vi "Keithley2612b_IV LOOP.vi"(3 "Error Query (False)":bool, 4 "Limit":dbl=1.0, 7 "Source Function (Current)":enum32{"Current", "Voltage"}(ring)=enum."Voltage", 8 "error in (no error)":errorcluster, 9 "Channel (Channel A)":T1, 10 "Node (0-64)":i8 min=0 max=64 step=1, 11 "VISA resource name":refnum<visa-resource-name>) -> (0 "error out":errorcluster)   [LabVIEW 2016]
doc: "This example shows how to configure the source and take a measurement."
uses:
  <instrlib>/Keithley 2600 Series/Public/Channel.ctl
  <vilib>/express/express shared/transition.llb/Dynamic To Waveform Array.vi
  <vilib>/express/express signal manip/GetorSetDDTAttributes/Set DDT Attributes/SetT0.vi
  <vilib>/express/express shared/transition.llb/Waveform Array To Dynamic.vi
  <vilib>/express/express signal manip/GetorSetDDTAttributes/Set DDT Attributes/Set DDT Properties.xnode
  <instrlib>/Keithley 2600 Series/Keithley 2600 Series.lvlib
panel:
  out "Current Number Past":dbl
  out "Voltage Output":string
  out "Current Output":string
  in  "Delay (s)":dbl
  in  "Step Size":dbl
  in  "End Voltage":dbl
  in  "Start Voltage":dbl
  # "(c) 2008 Keithley Instruments, Inc.  ALL RIGHTS RESERVED."
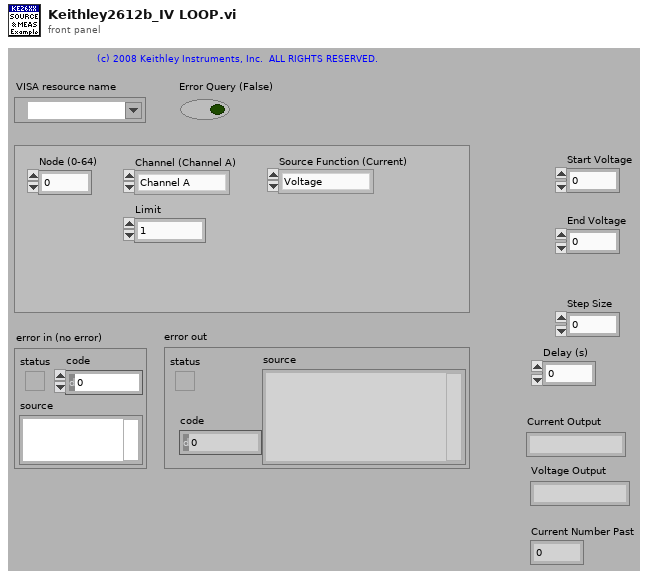
[diagram p1: front panel]
types:
  T1 = typedef "Keithley 2600 Series.lvlib/Channel.ctl" = enum32{"Channel A", "Channel B"}
  T2 = typedef "NI_Matrix.lvlib/RealMatrix.ctl" = dbl[][]
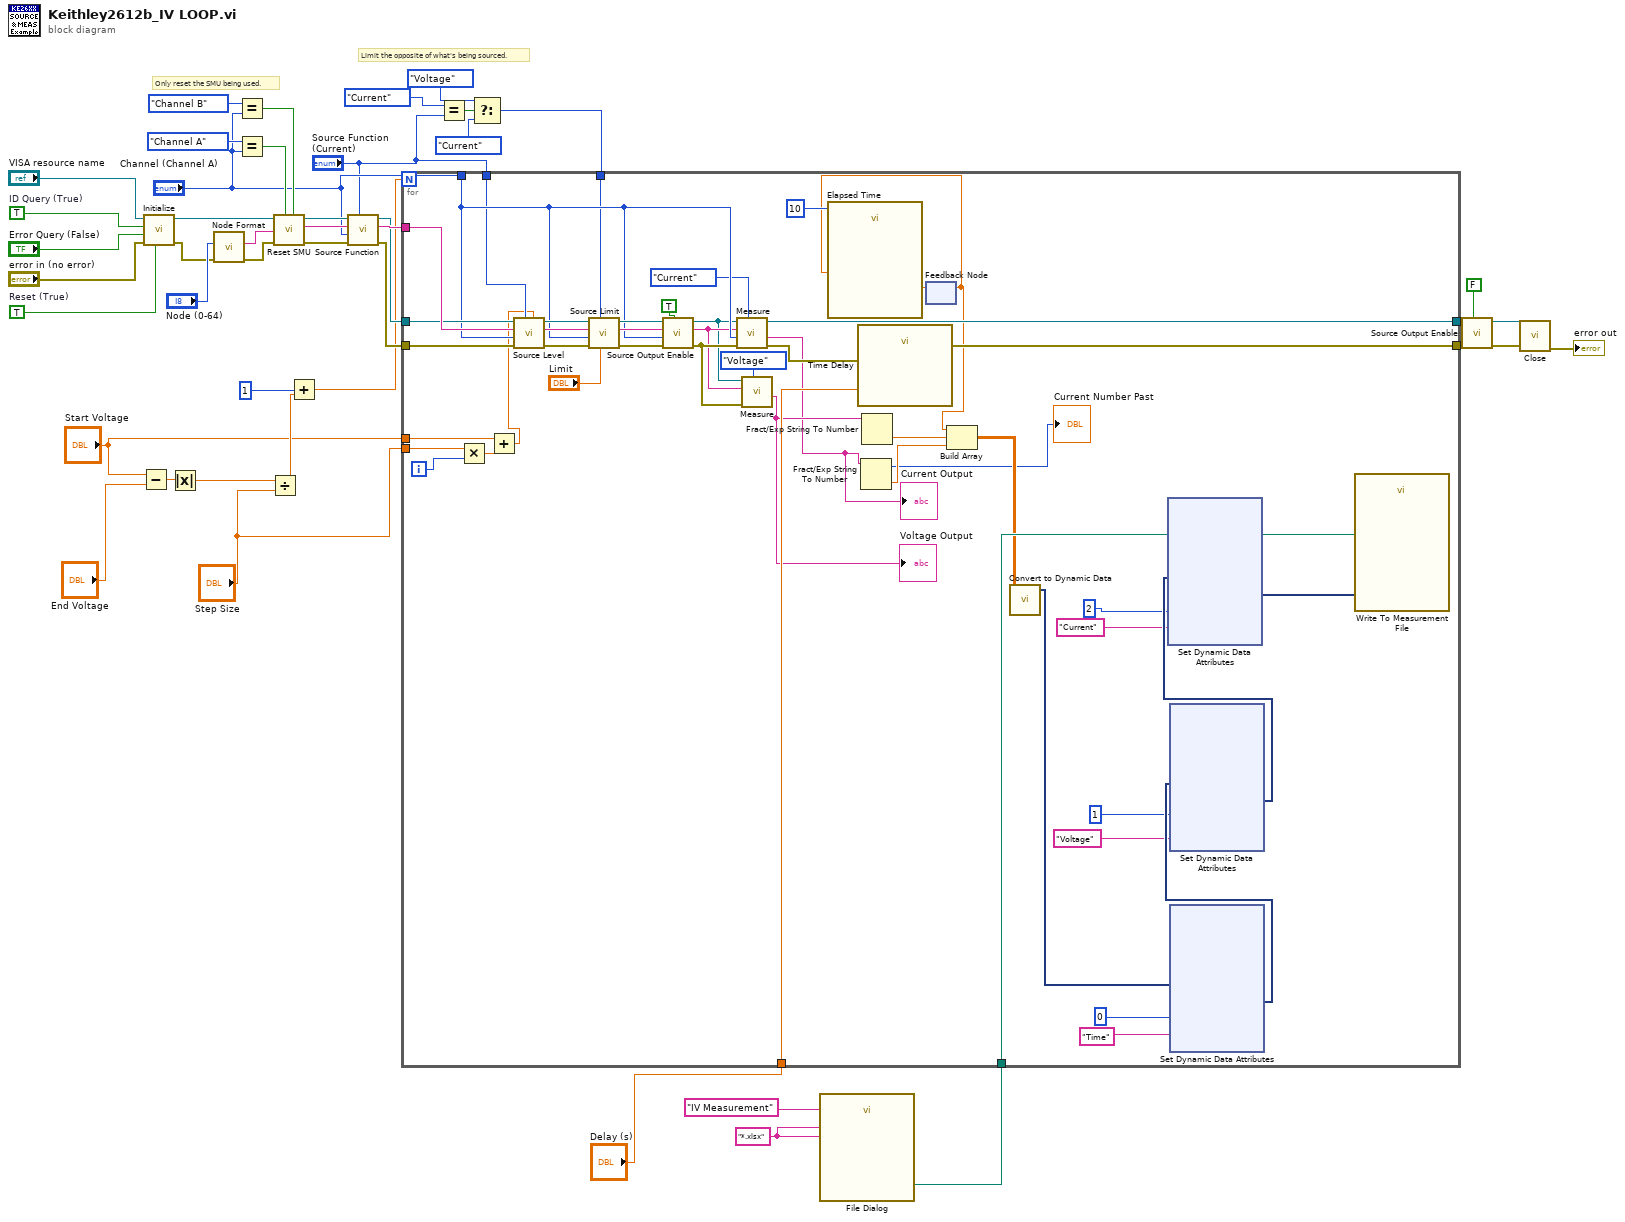
[diagram p0: block diagram]
diagram:
  w11 = "*.xlsx"
  w32 = TRUE  # Reset (True)
  w43 = TRUE  # ID Query (True)
  # "Limit the opposite of what's being sourced."
  # "Only reset the SMU being used."
  n1 = Subtract(x="Start Voltage", y="End Voltage") -> (x-y=w8:dbl)
  n2 = call <instrlib>:"Initialize.vi"("Reset (True)"=w32, "error in (no error)"="error in (no error)", "Error Query (False)"="Error Query (False)", "ID Query (True)"=w43, "VISA resource name"="VISA resource name") -> ("error out"=w1:errorcluster, "VISA resource name out"=w41:refnum<visa-resource-name>)  [unwired: 1 in, 4 out]
  n3 = Absolute Value(x=w8) -> (abs(x)=w7:dbl)
  n4 = call <instrlib>:"Node Format.vi"("error in"=w1, "Node (0-64)"="Node (0-64)") -> ("error out"=w28:errorcluster, "Formatted Node"=w29:string)  [unwired: 8 out]
  n5 = Equal?(x=enum32{"Channel A", "Channel B"}."Channel B", y="Channel (Channel A)") -> (x = y?=w37:bool)
  n6 = Equal?(x=enum32{"Channel A", "Channel B"}."Channel A", y="Channel (Channel A)") -> (x = y?=w38:bool)
  n7 = Divide(x=w7, y="Step Size") -> (x/y=w5:dbl)
  n8 = call <instrlib>:"Reset SMU.vi"("SMU B (No)"=w37, "SMU A (No)"=w38, "error in (no error)"=w28, "Node In"=w29, "VISA resource name"=w41) -> ("error out"=w36:errorcluster, "Node Out"=w34:string, "VISA resource name out"=w35:refnum<visa-resource-name>)  [unwired: 4 out]
  n9 = Add(x=1, y=w5) -> (x+y=w4:dbl)
  n10 = call <instrlib>:"Source Function.vi"("Function (Current)"="Source Function (Current)", "error in (no error)"=w36, "Channel (Channel A)"="Channel (Channel A)", "Node In"=w34, "VISA resource name"=w35) -> ("error out"=w26:errorcluster, "Node Out"=w25:string, "VISA resource name out"=w24:refnum<visa-resource-name>)  [unwired: 4 out]
  n11 = Equal?(x=enum32{"Current", "Voltage"}."Current", y="Source Function (Current)") -> (x = y?=w30:bool)
  n12 = Select(t=enum32{"Current", "Voltage"}."Voltage" ("x"), s=w30, f=enum32{"Current", "Voltage"}."Current") -> (s? t:f=w16:enum32{"Current", "Voltage"})
  n13 = call "File Dialog"("default name"="IV Measurement", "pattern (all files)"=w11, "pattern label"=w11) -> ("selected path"=w12:path)  [unwired: 9 in, 3 out]
  n14 = for {
    N: w4 -> [_]
    tunnel: w26 -> [w85]
    tunnel: w25 -> [w84]
    tunnel: w24 -> [w83]
    tunnel: "Channel (Channel A)" -> [w82]
    tunnel: "Source Function (Current)" -> [w78]
    tunnel: "Step Size" -> [w70]
    tunnel: "Start Voltage" -> [w79]
    tunnel: w16 -> [w77]
    tunnel: [w76] -> w14
    tunnel: [w73] -> w13
    tunnel: "Delay (s)" -> [w75]
    tunnel: w12 -> [w72]
    i -> [w81]
    n15 = Multiply(x=w70, y=w81) -> (x*y=w80:dbl)
    n16 = Add(x=w79, y=w80) -> (x+y=w56:dbl)
    n17 = call <instrlib>:"Source Level.vi"("Level (0.000)"=w56, "Function (Current)"=w78, "error in (no error)"=w85, "Channel (Channel A)"=w82, "Node In"=w84, "VISA resource name"=w83) -> ("error out"=w86:errorcluster, "Node Out"=w91:string, "VISA resource name out"=w87:refnum<visa-resource-name>)  [unwired: 3 out]
    n18 = call <instrlib>:"Source Limit.vi"("Limit (0.000)"="Limit", "Function (Current)"=w77, "error in (no error)"=w86, "Channel (Channel A)"=w82, "Node In"=w91, "VISA resource name"=w87) -> ("error out"=w89:errorcluster, "Node Out"=w92:string, "VISA resource name out"=w88:refnum<visa-resource-name>)  [unwired: 3 out]
    n19 = call <instrlib>:"Source Output Enable.vi"("Output (Off)"=TRUE, "error in (no error)"=w89, "Channel (Channel A)"=w82, "Node In"=w92, "VISA resource name"=w88) -> ("error out"=w68:errorcluster, "Node Out"=w67:string, "VISA resource name out"=w66:refnum<visa-resource-name>)  [unwired: 4 out]
    n20 = call <instrlib>:"Measure.vi"("Function (Current)"=enum32{"Current", "Voltage"}."Current" ("x"), "error in (no error)"=w68, "Channel (Channel A)"=w82, "Node In"=w67, "VISA resource name"=w66) -> ("error out"=w74:errorcluster, "Output"=w61:string, "VISA resource name out"=w76:refnum<visa-resource-name>)  [unwired: 2 in, 2 out]
    "Current Output" <- w61
    n21 = call <instrlib>:"Measure.vi"("Function (Current)"=enum32{"Current", "Voltage"}."Voltage" ("x"), "error in (no error)"=w68, "Node In"=w67, "VISA resource name"=w66) -> ("Output"=w63:string)  [unwired: 3 in, 4 out]
    "Voltage Output" <- w63
    n22 = call "Time Delay"("error in (no error)"=w74, "Delay Time (s)"=w75) -> ("error out"=w73:errorcluster)  [unwired: 9 in]
    n23 = Fract/Exp String To Number(string=w61) -> (offset past number=→"Current Number Past":i32, number=w60:dbl)  [unwired: 3 in]
    n24 = Fract/Exp String To Number(string=w63) -> (number=w62:dbl)  [unwired: 3 in, 1 out]
    n25 = feedback #1() -> (w57:dbl)  [unwired: 1 in]
    n26 = call "Elapsed Time"("Time Target (s)"=10, "Set Start Time (s)"=w57) -> ("Elapsed Time (s)"=w64:dbl)  [unwired: 10 in, 7 out]
    n27 = feedback-in #1(w64) -> ()
    n28 = Build Array(w57, w62, w60) -> (w71:T2)
    n29 = call "Convert to Dynamic Data"("2D Array"=w71) -> ("Dynamic Data Type"=w47:dynamicdata)  [unwired: 3 in]
    n30 = xnode "Set Dynamic Data Attributes"("Signals In"=w47, "Signal Index"=0, "Signal Name"="Time") -> ("Signals Out"=w54:dynamicdata)  [unwired: 1 in, 1 out]
    n31 = xnode "Set Dynamic Data Attributes"("Signals In"=w54, "Signal Index"=1, "Signal Name"="Voltage") -> ("Signals Out"=w55:dynamicdata)  [unwired: 1 in, 1 out]
    n32 = xnode "Set Dynamic Data Attributes"("Signals In"=w55, "Signal Index"=2, "Signal Name"="Current") -> ("Signals Out"=w46:dynamicdata)  [unwired: 1 in, 1 out]
    n33 = call "Write To Measurement File"("Signals"=w46, "Filename"=w72) -> ()  [unwired: 15 in, 3 out]
  }
  n34 = call <instrlib>:"Source Output Enable.vi"("Output (Off)"=FALSE, "error in (no error)"=w13, "VISA resource name"=w14) -> ("error out"=w17:errorcluster, "VISA resource name out"=w18:refnum<visa-resource-name>)  [unwired: 2 in, 5 out]
  n35 = call <instrlib>:"Close.vi"("error in (no error)"=w17, "VISA resource name"=w18) -> ("error out"=→"error out":errorcluster)  [unwired: 9 out]
